vi "WriteDigChan.vi"() -> ()   [LabVIEW 2017]
uses:
  Debug/WriteDigChan.dll
panel:
  out "data indicator":u8[](array[numeric])
  out "return type":i32
  in  "data":u8[](array[numeric])
  out "error out":errorcluster
  in  "error in (no error)":errorcluster
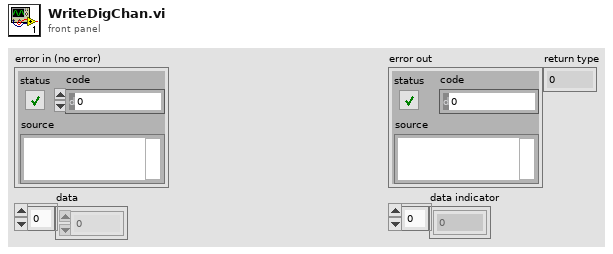
[diagram p1: front panel]
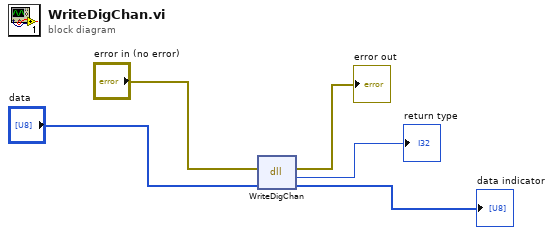
[diagram p0: block diagram]
diagram:
  n1 = dll-call lib="C:/Users/user/Documents/AyushWork/projects/WriteDigChan/WriteDigChan/Debug/WriteDigChan.dll" fn="WriteDigChan"(error in="error in (no error)", "data"="data") -> (error out=→"error out":errorcluster, "return type"=→"return type":i32, "data"=→"data indicator":u8[])  [unwired: 2 in, 1 out]
